vi "APDDSamp.vi"(0 "APD Data":dbl[][](array[numeric]), 1 "Data Period (s)":dbl, 2 "APD Disp. dSamp":i32, 3 "Time Stamp":timestamp) -> (14 "APD dSampd":waveform(dbl)[](array[waveform]))   [LabVIEW 2013]
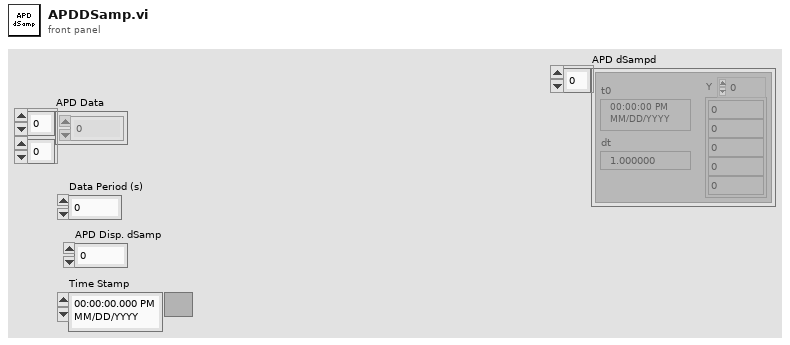
[diagram p1: front panel]
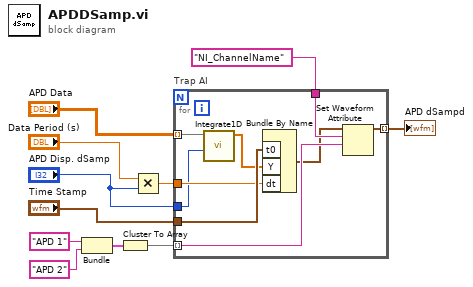
[diagram p0: block diagram]
diagram:
  n1 = Bundle("APD 1", "APD 2") -> (w1:cluster{string, string})  [unwired: 1 out]
  n2 = Cluster To Array(cluster=w1) -> (array=w3:string[])
  n3 = Multiply(x="Data Period (s)", y="APD Disp. dSamp") -> (x*y=w5:dbl)
  n4 = for "Trap AI" {
    tunnel: [w12] -> w8 mode=indexing
    tunnel: "Time Stamp" -> [w18]
    tunnel: "APD Disp. dSamp" -> [w15]
    tunnel: "APD Data" -> [w16] mode=indexing
    tunnel: w3 -> [w20] mode=indexing
    tunnel: "NI_ChannelName" ("name") -> [w19]
    tunnel: w5 -> [w17]
    n5 = call "Integrate1D.vi"("Avg N"=w15, "Array In"=w16) -> ("Array Out"=w14:dbl[])  [unwired: 9 in]
    n6 = Bundle By Name("t0"=w18, "Y"=w14, "dt"=w17) -> (w13:waveform(dbl))  [unwired: 1 out]
    n7 = Set Waveform Attribute(5:w20, 6:w19, 7:w13) -> (3:w12:waveform(dbl))  [unwired: 1 in, 2 out]
  }
  "APD dSampd" <- w8
